vi "P9374A Init for S.vi"(4 "Avg number":i32=1, 5 "points":i32=1, 6 "Port source to be off":string(combo)="2", 7 "ChannelParameter":string="S21", 8 "error in (no error)":errorcluster {"code" format="%.0x"}, 10 "Power dBm":dbl=-5.0, 11 "resource name":refnum<k15>="P9374A" caption="resource string") -> (0 "error out":errorcluster {"code" format="%.0x"}, 3 "instrument handle out":refnum<k15>)   [LabVIEW 2021]
uses:
  <instrlib>/Agilent NA/Agilent NA.lvlib
panel:
  in  "PortVal":i32=1 caption="power port" format="%.0g"
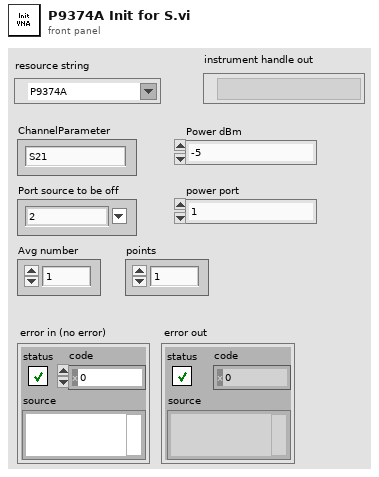
[diagram p1: front panel]
types:
  T1 = cluster{"ChannelNumber":i32, "WindowNumber":i32, "ChannelType":string, "ChannelParameter":string}
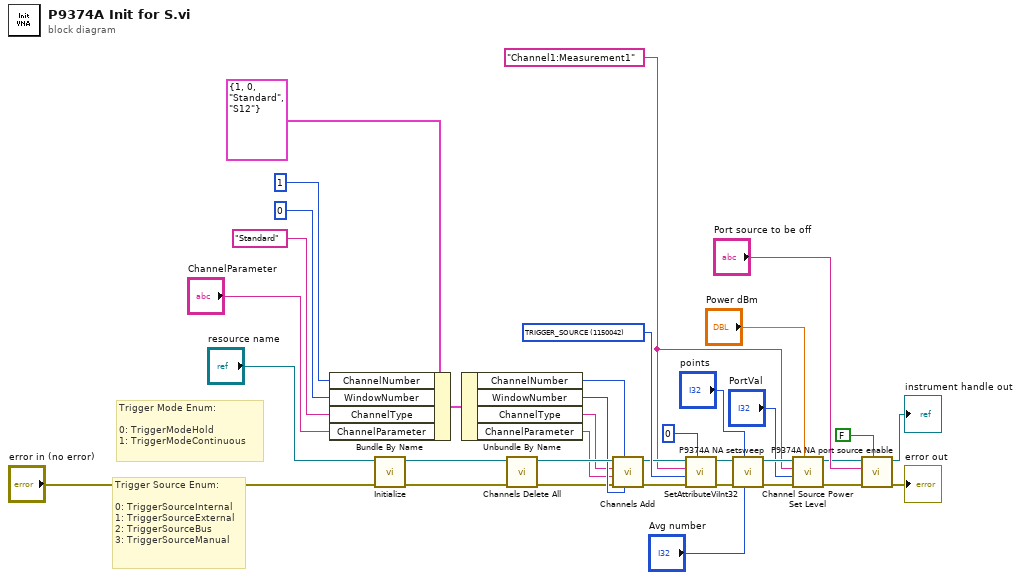
[diagram p0: block diagram]
diagram:
  w5 = "Channel1:Measurement1" ("RepCapIdentifier")
  w23 = u32 1150042 items=["CHANNEL_AVERAGING_FACTOR"=1150002, "CHANNEL_MEASUREMENT_ELECTRICAL_DELAY_MEDIUM"=1150178, "CHANNEL_MEASUREMENT_ELECTRICAL_DELAY_UNITS"=1150175, "CHANNEL_MEASUREMENT_FORMAT"=1150014, "CHANNEL_MEASUREMENT_LIMIT_NUMBER"=1150020, "CHANNEL_MEASUREMENT_TIME_DOMAIN_GATING_SHAPE"=1150140, "CHANNEL_MEASUREMENT_TIME_DOMAIN_GATING_TYPE"=1150144, "CHANNEL_MEASUREMENT_TIME_DOMAIN_PARAMETERS"=1150137, "CHANNEL_MEASUREMENT_TIME_DOMAIN_TRANSFORM_MODE"=1150147, "CHANNEL_MEASUREMENT_TRACE_MATH"=1150017, "CHANNEL_POINTS"=1150007, "CHANNEL_SWEEP_MODE"=1150009, "CHANNEL_SWEEP_TYPE"=1150012, "CHANNEL_TRIGGER_MODE"=1150013, "DISPLAY_ARRANGE_WINDOWS"=1150181, "SYSTEM_TIME_OUT_MILLISECONDS"=1150040, "TRIGGER_SOURCE"=1150042, "WINDOW_SIZE"=1150133, "WINDOW_TABLE"=1150134] ("AttributeID")
  # "Trigger Mode Enum:\n\n0: TriggerModeHold\n1: TriggerModeContinuous"
  # "Trigger Source Enum:\n\n0: TriggerSourceInternal\n1: TriggerSourceExternal\n2: TriggerSourceBus\n3: TriggerSourceManual"
  n1 = Bundle By Name(cluster=T1 {"ChannelNumber"=1, "WindowNumber"=0, "ChannelType"="Standard", "ChannelParameter"="S12"} ("Channel"), "ChannelNumber"=1, "WindowNumber"=0, "ChannelType"="Standard", "ChannelParameter"="ChannelParameter") -> (w14:T1)
  n2 = call <instrlib>:"Initialize.vi"("error in (no error)"="error in (no error)", "resource name"="resource name") -> ("error out"=w33:errorcluster, "instrument handle out"=w34:refnum<k15>)  [unwired: 8 in]
  n3 = Unbundle By Name(w14) -> ("ChannelNumber"=w31:i32, "WindowNumber"=w30:i32, "ChannelType"=w29:string, "ChannelParameter"=w28:string)
  n4 = call <instrlib>:"Channels Delete All.vi"("error in (no error)"=w33, "instrument handle"=w34) -> ("error out"=w27:errorcluster, "instrument handle out"=w32:refnum<k15>)  [unwired: 8 in]
  n5 = call <instrlib>:"Channels Add.vi"("WindowNumber"=w30, "ChannelNumber"=w31, "error in (no error)"=w27, "ChannelParameter"=w28, "ChannelType"=w29, "instrument handle"=w32) -> ("error out"=w21:errorcluster, "instrument handle out"=w22:refnum<k15>)  [unwired: 3 in, 1 out]
  n6 = call <instrlib>:"SetAttributeViInt32.vi"("AttributeValue"=0, "error in (no error)"=w21, "AttributeID"=w23, "RepCapIdentifier"=w5, "instrument handle"=w22) -> ("error out"=w24:errorcluster, "instrument handle out"=w25:refnum<k15>)  [unwired: 5 in]
  n7 = call "P9374A NA setsweep.vi"("Avg"="Avg number", "points"="points", "error in (no error)"=w24, "instrument handle"=w25) -> ("error out"=w6:errorcluster, "instrument handle out"=w7:refnum<k15>)  [unwired: 6 in]
  n8 = call <instrlib>:"Channel Source Power Set Level.vi"("Val"="Power dBm", "error in (no error)"=w6, "PortVal"="PortVal", "RepCapIdentifier"=w5, "instrument handle"=w7) -> ("error out"=w1:errorcluster, "instrument handle out"=w2:refnum<k15>)  [unwired: 5 in]
  n9 = call "P9374A NA port source enable.vi"("Enable"=FALSE, "error in (no error)"=w1, "Port"="Port source to be off", "instrument handle in"=w2) -> ("error out"=→"error out":errorcluster, "instrument handle out"=→"instrument handle out":refnum<k15>)  [unwired: 6 in]
